vi "create.SequencedUnitHeader.vi"(8 "error in (no error)":errorcluster, 10 "SequencedUnitHeader.Parms":T1={"Hdr Count"=0, "Hdr Unit"=0, "Hdr Sequence"=1, "Starting Sequence"=1}, 11 "SequencedUnitHeader in":refnum<class "SequencedUnitHeader.lvclass">) -> (0 "error out":errorcluster, 3 "SequencedUnitHeader out":refnum<class "SequencedUnitHeader.lvclass">)   [LabVIEW 2022 SP3, in "SequencedUnitHeader.lvclass"]
uses:
  SequencedUnitHeader.lvclass
  SequencedUnitHeader.Parameters.ctl
  FieldSpec.ctl
  SequencedUnitHeader.lvclass/SequencedUnitHeader.ctl
  PitchMessage/FieldValue.ctl
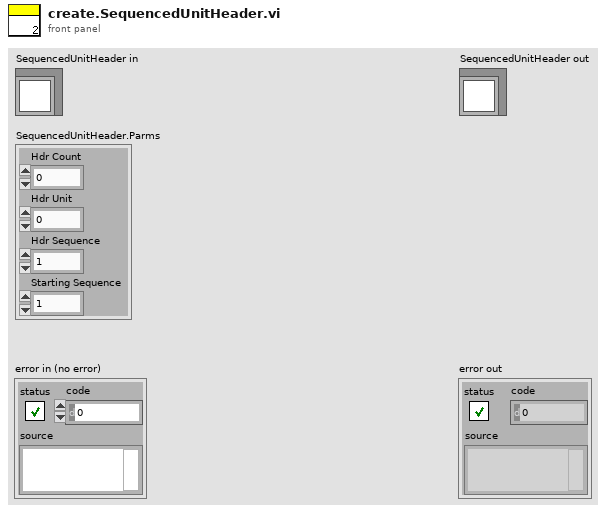
[diagram p1: front panel]
types:
  T1 = typedef "SequencedUnitHeader.lvclass/SequencedUnitHeader.Parameters.ctl" = cluster{"Hdr Count":u8, "Hdr Unit":u8, "Hdr Sequence":u32, "Starting Sequence":u32}
  T2 = typedef "FieldSpec.ctl" = cluster{"Name":string, "Offset":i32, "Length":i32, "FieldType":enum16{"Alphanumeric", "Binary", "BinaryLongPrice", "BinaryShortPrice", "BitField", "PrintableAscii", "Value"}}
  T3 = typedef "FieldValue.ctl" = variant
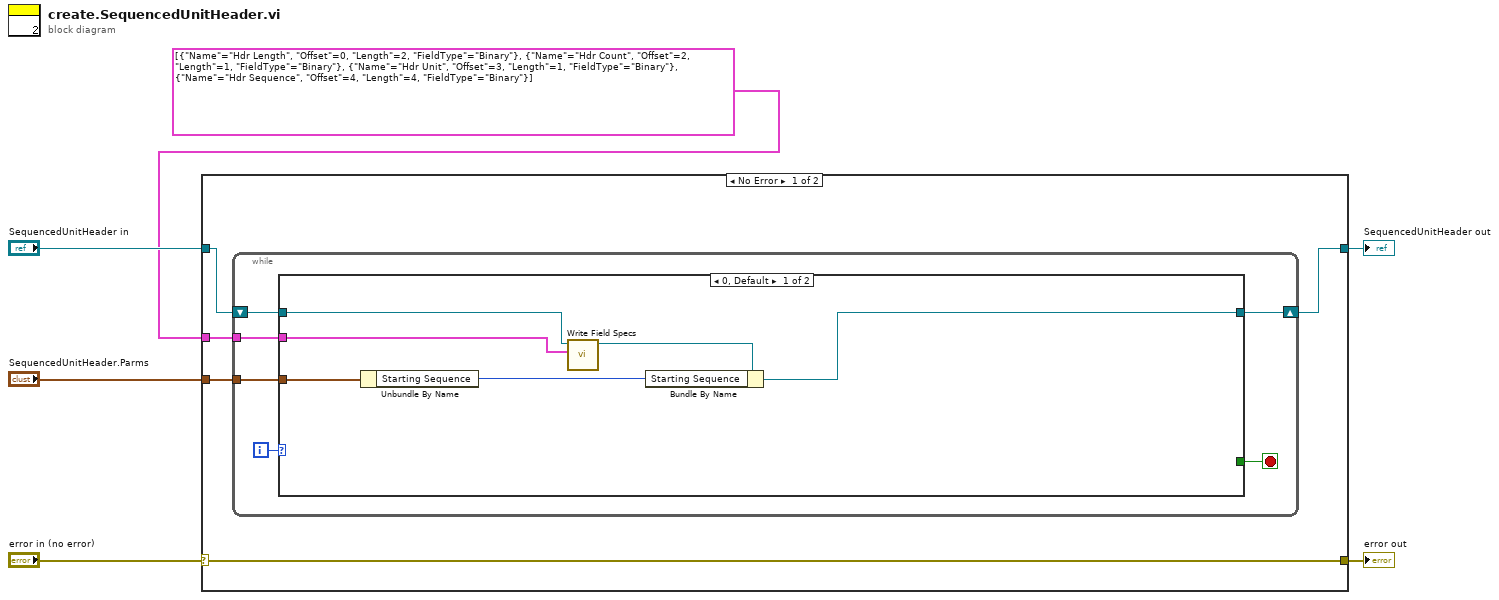
[diagram p0: block diagram]
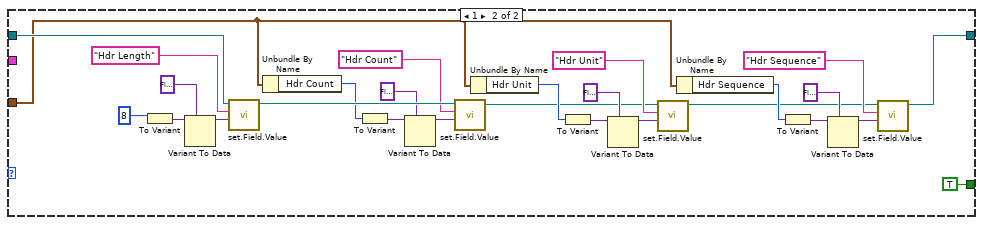
[diagram p2: hidden frame]
diagram:
  n1 = case shown="No Error" "error in (no error)" {
    selector: "error in (no error)" -> [w11 w52]
    tunnel: [w11 w52] -> w5
    tunnel: [w7 w51] -> w3
    tunnel: "SequencedUnitHeader in" -> [w8 w51]
    tunnel: T2[] [{"Name"="Hdr Length", "Offset"=0, "Length"=2, "FieldType"=enum."Binary"}, {"Name"="Hdr Count", "Offset"=2, "Length"=1, "FieldType"=enum."Binary"}, {"Name"="Hdr Unit", "Offset"=3, "Length"=1, "FieldType"=enum."Binary"}, {"Name"="Hdr Sequence", "Offset"=4, "Length"=4, "FieldType"=enum."Binary"}] ("appended array") -> [w10 _]
    tunnel: "SequencedUnitHeader.Parms" -> [w9 _]
    frame No Error {
      n2 = while {
        tunnel: w10 -> [w16]
        shift-right: [w14] -> w7
        shift-left: w8 -> [w15]
        tunnel: w9 -> [w12]
        i -> [w17]
        stop <- w13 stop-if-true
        n3 = case shown="0, Default" w17 {
          tunnel: [_ TRUE] -> w13
          tunnel: w16 -> [w23 _]
          tunnel: w15 -> [w22 w41]
          tunnel: [w18 w27] -> w14
          tunnel: w12 -> [w20 w25]
          frame 0, Default {
            n4 = Unbundle By Name(w20) -> ("Starting Sequence"=w19:u32)
            n5 = call-dynamic "Write Field Specs.vi"("Field Specs"=w23, "PitchMessage in"=w22) -> ("PitchMessage out"=w21:refnum<class "SequencedUnitHeader.lvclass">)  [unwired: 8 in, 1 out]
            n6 = Bundle By Name(cluster=w21, "Starting Sequence"=w19) -> (w18:refnum<class "SequencedUnitHeader.lvclass">)
          }
          frame 1 {
            n7 = To Variant(anything=u16 8) -> (Variant=w46:variant)
            n8 = Variant To Data(type=T3 variant ("FieldValue"), Variant=w46) -> (data=w47:T3)  [unwired: 1 in, 1 out]
            n9 = call-dynamic "set.Field.Value.vi"("Value"=w47, "FIeld.Name"="Hdr Length", "PitchMessage in"=w41) -> ("PitchMessage out"=w48:refnum<class "SequencedUnitHeader.lvclass">)  [unwired: 7 in, 1 out]
            n10 = Unbundle By Name(w25) -> ("Hdr Count"=w40:u8)
            n11 = To Variant(anything=w40) -> (Variant=w49:variant)
            n12 = Variant To Data(type=T3 variant ("FieldValue"), Variant=w49) -> (data=w50:T3)  [unwired: 1 in, 1 out]
            n13 = call-dynamic "set.Field.Value.vi"("Value"=w50, "FIeld.Name"="Hdr Count", "PitchMessage in"=w48) -> ("PitchMessage out"=w34:refnum<class "SequencedUnitHeader.lvclass">)  [unwired: 7 in, 1 out]
            n14 = Unbundle By Name(w25) -> ("Hdr Unit"=w35:u8)
            n15 = To Variant(anything=w35) -> (Variant=w38:variant)
            n16 = Variant To Data(type=T3 variant ("FieldValue"), Variant=w38) -> (data=w39:T3)  [unwired: 1 in, 1 out]
            n17 = call-dynamic "set.Field.Value.vi"("Value"=w39, "FIeld.Name"="Hdr Unit", "PitchMessage in"=w34) -> ("PitchMessage out"=w28:refnum<class "SequencedUnitHeader.lvclass">)  [unwired: 7 in, 1 out]
            n18 = Unbundle By Name(w25) -> ("Hdr Sequence"=w29:u32)
            n19 = To Variant(anything=w29) -> (Variant=w32:variant)
            n20 = Variant To Data(type=T3 variant ("FieldValue"), Variant=w32) -> (data=w33:T3)  [unwired: 1 in, 1 out]
            n21 = call-dynamic "set.Field.Value.vi"("Value"=w33, "FIeld.Name"="Hdr Sequence", "PitchMessage in"=w28) -> ("PitchMessage out"=w27:refnum<class "SequencedUnitHeader.lvclass">)  [unwired: 7 in, 1 out]
          }
        }
      }
    }
    frame Error {
    }
  }
  "error out" <- w5
  "SequencedUnitHeader out" <- w3
